vi "销售明细生成excel(子VI).vi"(10 "appended path":path, 11 "数组":string[](array[string])) -> ()   [LabVIEW 2013]
uses:
  <vilib>/Utility/file.llb/Write To Spreadsheet File (string).vi
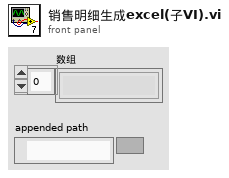
[diagram p1: front panel]
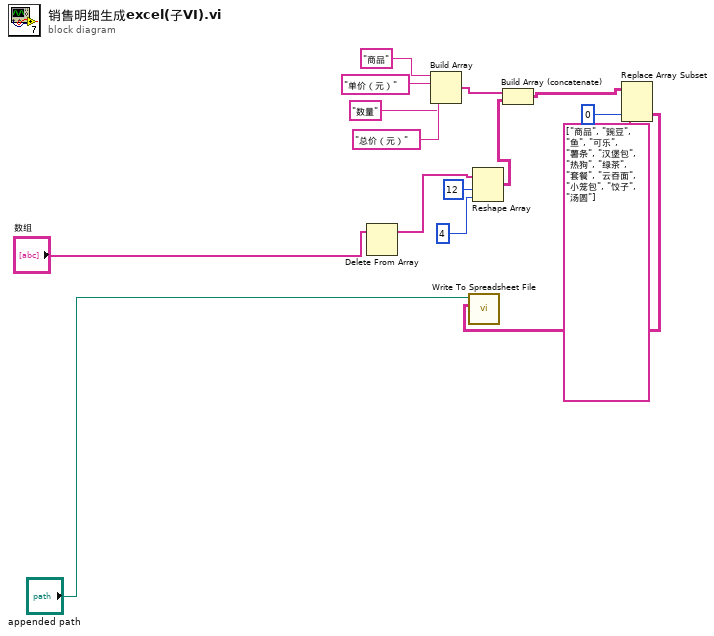
[diagram p0: block diagram]
diagram:
  n1 = Delete From Array "Delete From Array"(array="数组") -> (array with subset deleted=w4:string[])  [unwired: 2 in, 1 out]
  n2 = Build Array("商品" ("元素"), "单价（元）", "数量" ("元素"), "总价（元）" ("元素")) -> (w9:string[])
  n3 = Reshape Array(w4, 12 ("维数大小"), 4 ("维数大小")) -> (w10:string[][])
  n4 = Build Array (concatenate)(w9, w10) -> (w12:string[][])
  n5 = Replace Array Subset(array=w12, new element=string[] ["商品", "豌豆", "鱼", "可乐", "薯条", "汉堡包", "热狗", "绿茶", "套餐", "云吞面", "小笼包", "饺子", "汤圆"] ("新元素/子数组"), index (col)=0 ("禁用的索引 (列)")) -> (w14:string[][])  [unwired: 1 in]
  n6 = call-poly <vilib>:"Write To Spreadsheet File.vi"("2D data"=w14, "file path (dialog if empty)"="appended path") -> ()  [unwired: 4 in, 3 out]
